vi "Periodic Tasks.vi"(8 "error in":errorcluster) -> ()   [LabVIEW 2016]
doc: "This VI runs in parallel to other tasks. It can contain as many user-defined periodic loops as you need. These can carry out PID or other sorts of timed response."
uses:
  <vilib>/Rock Robotics/WPI/Solenoid/WPI_SolenoidValue.ctl
  dash_to_rio_cluster.ctl
  Shifter override.ctl
  Robot Global Data.vi
  <vilib>/Rock Robotics/WPI/Solenoid/WPI_SolenoidSetEnum.vi
  <vilib>/Rock Robotics/Network Tables/NT Read String.vi
  <vilib>/Rock Robotics/Network Tables/NT Write String.vi
  Senor Drivers-Libs/ADIS16448-LabVIEW_libs/ADI MXP IMU/FRC_ADIS16448_IMU.lvlib
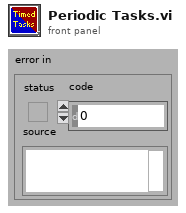
[diagram p1: front panel]
types:
  T1 = typedef "dash_to_rio_cluster.ctl" = cluster{"Left drive PID ":cluster{"P":dbl, "I":dbl, "D":dbl, "F":dbl}, "Right drive PID ":cluster{"P":dbl, "I":dbl, "D":dbl, "F":dbl}, "Shooter drive PID ":cluster{"P":dbl, "I":dbl, "D":dbl, "F":dbl}, "Shifter override":T2, "Reset gyro?":bool}
  T2 = typedef "Shifter override.ctl" = enum16{"No override", "High ", "Low"}
  T3 = typedef "WPI_SolenoidValue.ctl" = enum16{"Off", "On", "Forward", "Reverse"}
  T4 = typedef "FRC_ADIS16448_IMU.lvlib/WPI_IMU_ADIS16448_InterruptDevRef.ctl" = cluster{"ADI IMU DevRef":T5, "InterruptRef":T7}
  T5 = typedef "FRC_ADIS16448_IMU.lvlib/WPI_IMU_ADIS16448_IMUDevRef.ctl" = cluster{"DevStatus":errorcluster, "Handle":i32, "SPI Bus":T6, "Device Found":bool, "Device Ready":bool, "Yaw Axis":enum16{"X", "Y", "Z"}, "AHRS Algorithm":enum16{"Complementary", "Madgwick"}, "Serial":u16, "Lot ID 2":u16, "Lot ID 1":u16, "Product ID":u16}
  T6 = typedef "spi_bus.ctl" = enum16{"SPI On-Board, CS0", "SPI On-Board, CS1", "SPI On-Board, CS2", "SPI On-Board, CS3", "SPI MXP", "Invalid"}
  T7 = typedef "WPI_InterruptRef.ctl" = cluster{"DevStatus":errorcluster, "InterruptIndex":T8}
  T8 = typedef "FPGA_InterruptIndex.ctl" = enum8{"0", "1", "2", "3", "4", "5", "6", "7", "Invalid"}
  T9 = typedef "WPI_MotorControlDeviceRef.ctl" = cluster{"DeviceStatus":errorcluster, "Type":T10, "PWM":cluster{"PWM Channel":T11, "DeadBand":T12}, "CAN":cluster{"Device Number":u8, "SetOutput VI Ref":variant, "GetOutput VI Ref":variant, "Enable VI Ref":variant, "Disable VI Ref":variant, "Data":variant}, "Invert":bool}
  T10 = typedef "WPI_MotorControlType.ctl" = enum16{"PWM", "CAN"}
  T11 = typedef "FPGA_DIOPWMChannel.ctl" = enum8{"PWM 0", "PWM 1", "PWM 2", "PWM 3", "PWM 4", "PWM 5", "PWM 6", "PWM 7", "PWM 8", "PWM 9", "PWM MXP 0", "PWM MXP 1", "PWM MXP 2", "PWM MXP 3", "PWM MXP 4", "PWM MXP 5", "PWM MXP 6", "PWM MXP 7", "PWM MXP 8", "PWM MXP 9", "Invalid"}
  T12 = typedef "WPI_PWMDeadband.ctl" = cluster{"Name":string, "maxPositivePwm":i32, "minPositivePwm":i32, "centerPwm":i32, "maxNegativePwm":i32, "minNegativePwm":i32, "angularRange":u16}
  T13 = typedef "WPI_CANTalonSRX_GlobalStatus.ctl" = cluster{"Applied Throttle":dbl, "Module Enabled":bool, "CAN Error":errorcluster, "Closed Loop Error":dbl, "Forward Limit Switch Closed":bool, "Reverse Limit Switch Closed":bool, "Sensor Position":dbl, "Sensor Velocity":dbl, "Current":dbl, "Sticky Fault - Over Temp":bool, "Sticky Fault - Under Voltage":bool, "Sticky Fault - Forward Limit":bool, "Sticky Fault - Reverse Limit":bool, "Sticky Fault - Forward Soft Limit":bool, "Sticky Fault - Reverse Soft Limit":bool, "Brake is Enabled":bool, "Encoder Position":dbl, "Encoder Velocity":dbl, "Encoder Index Count":dbl, "Encoder A Pin State":bool, "Encoder B Pin State":bool, "Encoder Index Pin State":bool, "Analog In":dbl, "Analog In Velocity":dbl, "Temperature (C)":dbl, "Battery Voltage":dbl, "Control 5 Is Supported":bool, "Current Profile Slot Select":dbl, "Pos Div 8":bool, "Vel Div 4":bool, "Pulse Width Position":i32, "Pulse Width Velocity":i32, "Pulse Width Rise To Rise (us)":i32, "Pulse Width Rise To Fall (us)":i32, "Mot Prof Active Is Under Run":bool, "Mot Prof Active Has Under Run":bool, "Mot Prof Active Is Last":bool, "Mot Prof Active Velocity Only":bool, "Mot Prof Active Is Valid":bool, "Mot Prof Buffer Is Full":bool, "Mot Prof Active Profile Slot Select":i32, "Mot Prof NextID":i32, "Mot Prof Count":i32, "Mot Prof Active Velocity":dbl, "Mot Prof Active Position":dbl, "Mot Prof Output Enable":i32}
  T14 = cluster{"Gear status":cluster{"Gear at bottom?":bool, "Gear at top?":bool}, "Drive train current":cluster{"Left current":dbl, " Right current":dbl}, "Total robot current":dbl, "Gyro angle":dbl, "Shooter Wheel speed":dbl, "Climber current":dbl}
  T15 = typedef "WPI_SolenoidDevRef.ctl" = cluster{"DevStatus":errorcluster, "Pneumatics Control Module":u8, "Forward Solenoid Channel":T16, "Reverse Solenoid Channel":T16}
  T16 = typedef "WPI_SolenoidChannel.ctl" = enum8{"Solenoid 0", "Solenoid 1", "Solenoid 2", "Solenoid 3", "Solenoid 4", "Solenoid 5", "Solenoid 6", "Solenoid 7", "Invalid"}
  T17 = cluster{"Y":dbl, "X":dbl, "Left out":dbl, "Right out":dbl}
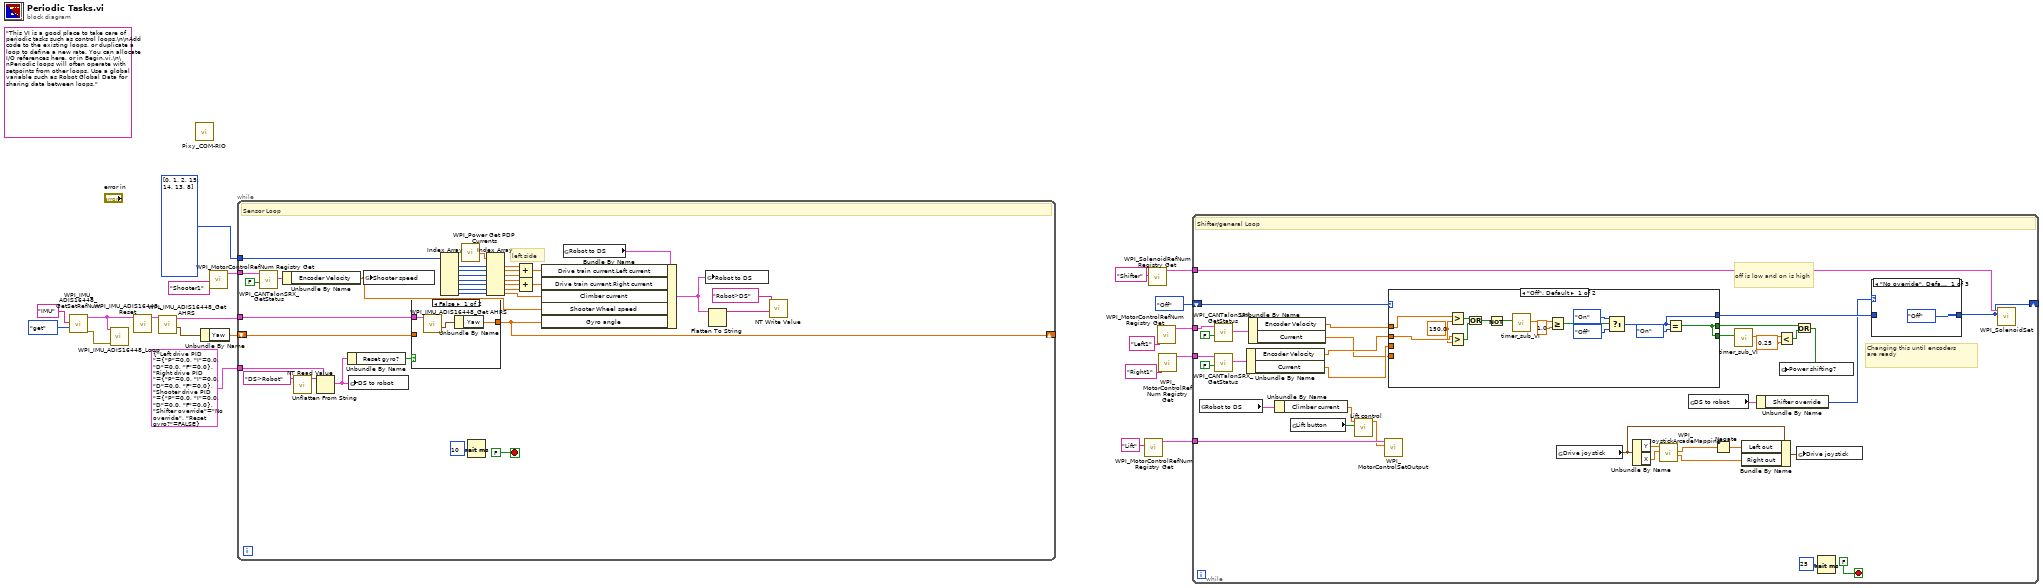
[diagram p0: block diagram]
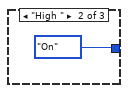
[diagram p2: hidden frame]
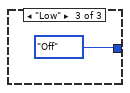
[diagram p3: hidden frame]
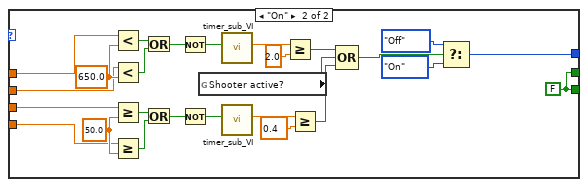
[diagram p4: hidden frame]
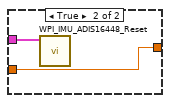
[diagram p5: hidden frame]
diagram:
  (unwired) "This VI is a good place to take care of periodic tasks such as control loops.\n\nAdd code to the existing loops, or duplicate a loop to define a new rate. You can allocate I/O references here, or in Begin.vi.\n\nPeriodic loops will often operate with setpoints from other loops. Use a global variable such as Robot Global Data for sharing data between loops."
  n1 = call "WPI_IMU_ADIS16448_GetSetRefNum.vi"("menu"=enum16{"set", "get"}."get", "refnum name"="IMU") -> ("error out"=w4:errorcluster, "ADI IMU Interrupt DevRef Get"=w5:T4)  [unwired: 8 in]
  n2 = call "WPI_IMU_ADIS16448_Loop.vi"("error in"=w4, "ADI IMU Interrupt DevRef"=w5) -> ()  [unwired: 8 in, 2 out]
  n3 = call "WPI_IMU_ADIS16448_Reset.vi"("ADI IMU Interrupt DevRef"=w5) -> ("ADI IMU Interrupt DevRef Out"=w3:T4)  [unwired: 9 in, 1 out]
  n4 = call "WPI_IMU_ADIS16448_Get AHRS.vi"("ADI IMU Interrupt DevRef"=w3) -> ("IMU AHRS Delta Out"=w1:cluster{"Pitch":dbl, "Roll":dbl, "Yaw":dbl}, "ADI IMU Interrupt DevRef"=w2:T4)  [unwired: 6 in, 3 out]
  n5 = call "Pixy_COM-RIO.vi"() -> ()  [unwired: 11 in]
  n6 = Unbundle By Name(w1) -> ("Yaw"=w6:dbl)
  n7 = call <vilib>:"WPI_MotorControlRefNum Registry Get.vi"("refnum name"="Shooter1") -> ("MotorControlDevRef"=w18:T9)  [unwired: 9 in, 1 out]
  n8 = while "Sensor Loop" {
    tunnel: w2 -> [w56]
    tunnel: w18 -> [w53]
    tunnel: i32[] [0, 1, 2, 15, 14, 13, 8] -> [w32]
    tunnel: T1 {"Left drive PID "={"P"=0.0, "I"=0.0, "D"=0.0, "F"=0.0}, "Right drive PID "={"P"=0.0, "I"=0.0, "D"=0.0, "F"=0.0}, "Shooter drive PID "={"P"=0.0, "I"=0.0, "D"=0.0, "F"=0.0}, "Shifter override"=enum."No override", "Reset gyro?"=FALSE} ("DS to robot") -> [w26]
    shift-right: [w22] -> _
    shift-left: w6 -> [w23]
    stop <- FALSE stop-if-true
    # "left side"
    # "Sensor Loop"
    n9 = call <vilib>:"WPI_CANTalonSRX_GetStatus.vi"("Clear Sticky Faults"=FALSE, "CAN Talon SRX Ref"=w53) -> ("Talon SRX Status"=w54:T13)  [unwired: 7 in, 2 out]
    n10 = Unbundle By Name(w54) -> ("Encoder Velocity"=w31:dbl)
    n11 = call-poly <vilib>:"NT Read Value.vi"("Name"="DS>Robot") -> ("String"=w27:string)  [unwired: 9 in, 1 out]
    n12 = Unflatten From String(type=w26, binary string=w27) -> (value=w25:T1)  [unwired: 3 in, 2 out]
    n13 = Unbundle By Name(w25) -> ("Reset gyro?"=w24:bool)
    n14 = global write "Robot Global Data.vi" "DS to robot"(w25) -> ()
    n15 = global write "Robot Global Data.vi" "Shooter speed"(w31) -> ()
    n16 = case shown="False" w24 {
      tunnel: w56 -> [w59 w61]
      tunnel: [w60 w62] -> w22
      tunnel: w23 -> [_ w62]
      frame False {
        n17 = call "WPI_IMU_ADIS16448_Get AHRS.vi"("ADI IMU Interrupt DevRef"=w59) -> ("IMU AHRS Delta Out"=w58:cluster{"Pitch":dbl, "Roll":dbl, "Yaw":dbl})  [unwired: 6 in, 4 out]
        n18 = Unbundle By Name(w58) -> ("Yaw"=w60:dbl)
      }
      frame True {
        n19 = call "WPI_IMU_ADIS16448_Reset.vi"("ADI IMU Interrupt DevRef"=w61) -> ()  [unwired: 9 in, 2 out]
      }
    }
    n20 = Index Array(array=w32) -> (element #1=w38:i32, element #2=w37:i32, element #3=w36:i32, element #4=w35:i32, element #5=w34:i32, element #6=w33:i32, element #7=w30:i32)  [unwired: 7 in]
    n21 = call <vilib>:"WPI_Power Get PDP Currents.vi"() -> ("all currents (A)"=w49:dbl[])  [unwired: 13 in, 2 out]
    n22 = Wait (ms)(milliseconds to wait=u32 10) -> ()  [unwired: 1 out]
    n23 = Index Array(array=w49, index #1=w38, index #2=w37, index #3=w36, index #4=w35, index #5=w34, index #6=w33, index #7=w30) -> (element #1=w48:dbl, element #2=w47:dbl, element #3=w46:dbl, element #4=w45:dbl, element #5=w44:dbl, element #6=w43:dbl, element #7=w29:dbl)
    n24 = Compound Arithmetic op=ADD(w48, w47, w46) -> (w42:dbl)
    n25 = Compound Arithmetic op=ADD(w45, w44, w43) -> (w41:dbl)
    n26 = global read "Robot Global Data.vi" "Robot to DS"() -> (w40:T14)
    n27 = Bundle By Name(cluster=w40, "Drive train current.Left current"=w42, "Drive train current.Right current"=w41, "Climber current"=w29, "Shooter Wheel speed"=w31, "Gyro angle"=w22) -> (w39:T14)
    n28 = global write "Robot Global Data.vi" "Robot to DS"(w39) -> ()
    n29 = Flatten To String(anything=w39) -> (data string=w51:string)  [unwired: 3 in, 2 out]
    n30 = call-poly <vilib>:"NT Write Value.vi"("String"=w51, "Name"="Robot>DS") -> ()  [unwired: 9 in, 1 out]
  }
  n31 = call <vilib>:"WPI_MotorControlRefNum Registry Get.vi"("refnum name"="Lift") -> ("MotorControlDevRef"=w8:T9)  [unwired: 9 in, 1 out]
  n32 = call <vilib>:"WPI_SolenoidRefNum Registry Get.vi"("refnum name"="Shifter") -> ("SolenoidDevRef"=w15:T15)  [unwired: 9 in, 1 out]
  n33 = call <vilib>:"WPI_MotorControlRefNum Registry Get.vi"("refnum name"="Left1") -> ("MotorControlDevRef"=w11:T9)  [unwired: 9 in, 1 out]
  n34 = call <vilib>:"WPI_MotorControlRefNum Registry Get.vi"("refnum name"="Right1") -> ("MotorControlDevRef"=w10:T9)  [unwired: 9 in, 1 out]
  n35 = while "Shifter Loop" {
    shift-right: [w65] -> _
    shift-left: WPI_SolenoidValue."Off" ("Value") -> [w96]
    tunnel: w15 -> [w90]
    tunnel: w11 -> [w79]
    tunnel: w10 -> [w78]
    tunnel: w8 -> [w72]
    stop <- FALSE stop-if-true
    # "Changing this until encoders\nare ready"
    # "off is low and on is high"
    # "Shifter/general Loop"
    n36 = global read "Robot Global Data.vi" "Robot to DS"() -> (w70:T14)
    n37 = call <vilib>:"WPI_CANTalonSRX_GetStatus.vi"("Clear Sticky Faults"=FALSE, "CAN Talon SRX Ref"=w79) -> ("Talon SRX Status"=w83:T13)  [unwired: 7 in, 2 out]
    n38 = call <vilib>:"WPI_CANTalonSRX_GetStatus.vi"("Clear Sticky Faults"=FALSE, "CAN Talon SRX Ref"=w78) -> ("Talon SRX Status"=w81:T13)  [unwired: 7 in, 2 out]
    n39 = Unbundle By Name(w81) -> ("Encoder Velocity"=w76:dbl, "Current"=w75:dbl)
    n40 = Unbundle By Name(w83) -> ("Encoder Velocity"=w77:dbl, "Current"=w74:dbl)
    n41 = Unbundle By Name(w70) -> ("Climber current"=w68:dbl)
    n42 = global read "Robot Global Data.vi" "Lift button"() -> (w69:bool)
    n43 = call "Lift control.vi"("Lift button?"=w69, "Lift Current"=w68) -> ("Lift power"=w71:dbl)  [unwired: 9 in]
    n44 = call <vilib>:"WPI_MotorControlSetOutput.vi"("Output"=w71, "MotorControlDevRef"=w72) -> ()  [unwired: 7 in, 3 out]
    n45 = case shown="\"Off\", Default" w96 {
      tunnel: w77 -> [w116 w133]
      tunnel: w76 -> [w115 w132]
      tunnel: [w104 w118] -> w66
      tunnel: w75 -> [_ w123]
      tunnel: w74 -> [_ w124]
      tunnel: [w102 w117] -> w93
      tunnel: [w102 w117] -> w91
      frame "Off", Default {
        w114 = 150.0 ("y")
        n46 = Greater?(x=w116, y=w114) -> (0:w113:bool)
        n47 = Greater?(x=w115, y=w114) -> (0:w112:bool)
        n48 = Or(x=w113, y=w112) -> (x .or. y?=w108:bool)
        n49 = Not(x=w108) -> (.not. x?=w109:bool)
        n50 = call "timer_sub_VI.vi"("Reset"=w109) -> ("Time (Secs)"=w107:dbl)  [unwired: 10 in]
        n51 = Greater Or Equal?(x=w107, y=1.0) -> (x >= y?=w105:bool)
        n52 = Select(t=WPI_SolenoidValue."On" ("Value"), s=w105, f=WPI_SolenoidValue."Off" ("Value")) -> (s? t:f=w104:T3)
        n53 = Equal?(x=w104, y=WPI_SolenoidValue."On") -> (x = y?=w102:bool)
      }
      frame "On" {
        w117 = FALSE
        w131 = 50.0 ("y")
        w142 = 650.0 ("y")
        n54 = Less?(x=w133, y=w142) -> (x < y?=w141:bool)
        n55 = Less?(x=w132, y=w142) -> (x < y?=w140:bool)
        n56 = Greater Or Equal?(x=w123, y=w131) -> (x >= y?=w130:bool)
        n57 = Greater Or Equal?(x=w124, y=w131) -> (x >= y?=w129:bool)
        n58 = Or(x=w141, y=w140) -> (x .or. y?=w136:bool)
        n59 = Or(x=w130, y=w129) -> (x .or. y?=w127:bool)
        n60 = Not(x=w136) -> (.not. x?=w137:bool)
        n61 = Not(x=w127) -> (.not. x?=w128:bool)
        n62 = global read "Robot Global Data.vi" "Shooter active?"() -> (w120:bool)
        n63 = call "timer_sub_VI.vi"("Reset"=w137) -> ("Time (Secs)"=w135:dbl)  [unwired: 10 in]
        n64 = call "timer_sub_VI.vi"("Reset"=w128) -> ("Time (Secs)"=w126:dbl)  [unwired: 10 in]
        n65 = Greater Or Equal?(x=w135, y=2.0) -> (x >= y?=w121:bool)
        n66 = Greater Or Equal?(x=w126, y=0.4) -> (x >= y?=w119:bool)
        n67 = Compound Arithmetic op=OR(w121, w120, w119) -> (w122:bool)
        n68 = Select(t=WPI_SolenoidValue."Off" ("Value"), s=w122, f=WPI_SolenoidValue."On" ("Value")) -> (s? t:f=w118:T3)
      }
    }
    n69 = global read "Robot Global Data.vi" "Drive joystick"() -> (w86:T17)
    n70 = Unbundle By Name(w86) -> ("Y"=w89:dbl, "X"=w88:dbl)
    n71 = call <vilib>:"WPI_JoystickArcadeMapping.vi"("Y axis value"=w89, "X axis value"=w88) -> ("Right Motor Value"=w84:dbl, "Left Motor Value"=w85:dbl)  [unwired: 8 in]
    n72 = global read "Robot Global Data.vi" "DS to robot"() -> (w67:T1)
    n73 = Negate(x=w85) -> (-x=w63:dbl)
    n74 = call "timer_sub_VI.vi"("Reset"=w91) -> ("Time (Secs)"=w94:dbl)  [unwired: 10 in]
    n75 = Bundle By Name(cluster=w86, "Left out"=w63, "Right out"=w84) -> (w87:T17)
    n76 = Unbundle By Name(w67) -> ("Shifter override"=w64:T2)
    n77 = Less?(x=w94, y=0.25) -> (x < y?=w92:bool)
    n78 = Or(x=w93, y=w92) -> (x .or. y?=w73:bool)
    n79 = global write "Robot Global Data.vi" "Power shifting?"(w73) -> ()
    n80 = global write "Robot Global Data.vi" "Drive joystick"(w87) -> ()
    n81 = Wait (ms)(milliseconds to wait=u32 25) -> ()  [unwired: 1 out]
    n82 = case shown="\"No override\", Default" w64 {
      tunnel: w66 -> [_ _ _]
      tunnel: [WPI_SolenoidValue."Off" ("Value") WPI_SolenoidValue."On" ("Value") WPI_SolenoidValue."Off" ("Value")] -> w65
      frame "No override", Default {
      }
      frame "High " {
      }
      frame "Low" {
      }
    }
    n83 = call-poly <vilib>:"WPI_SolenoidSet.vi"("Value"=w65, "SolenoidDevRef"=w90) -> ()  [unwired: 8 in, 2 out]
  }
